vi "充电数据解析(81).vi"(1 "充电数据解析(81)":dbl[](array[numeric])) -> (0 "充电状态":string[](array[string]))   [LabVIEW 2013]
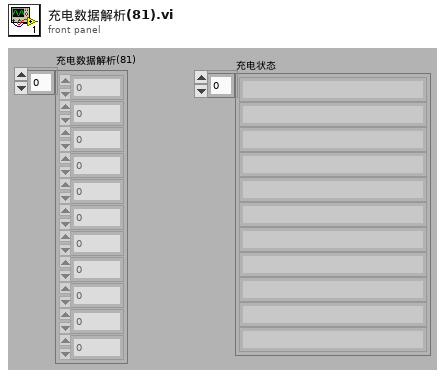
[diagram p1: front panel]
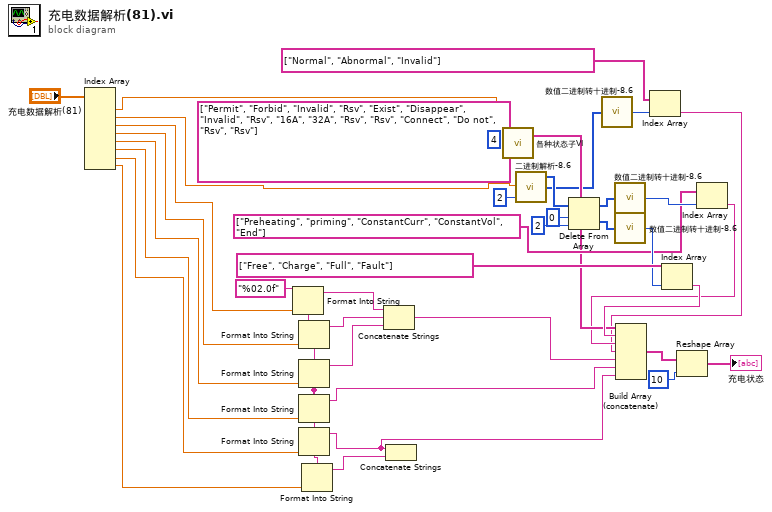
[diagram p0: block diagram]
diagram:
  w32 = "%02.0f" ("格式字符串")
  n1 = Index Array(array="充电数据解析(81)") -> (element #1=w12:dbl, element #2=w11:dbl, element #3=w10:dbl, element #4=w9:dbl, element #5=w8:dbl, element #6=w7:dbl, element #7=w6:dbl, element #8=w5:dbl)  [unwired: 8 in]
  n2 = Format Into String(format string=w32, w10) -> (resulting string=w33:string)  [unwired: 2 in, 1 out]
  n3 = Format Into String(format string=w32, w9) -> (resulting string=w34:string)  [unwired: 2 in, 1 out]
  n4 = Format Into String(format string=w32, w8) -> (resulting string=w35:string)  [unwired: 2 in, 1 out]
  n5 = Format Into String(format string=w32, w7) -> (resulting string=w38:string)  [unwired: 2 in, 1 out]
  n6 = Format Into String(format string=w32, w6) -> (resulting string=w39:string)  [unwired: 2 in, 1 out]
  n7 = Format Into String(format string=w32, w5) -> (resulting string=w36:string)  [unwired: 2 in, 1 out]
  n8 = Concatenate Strings(w33, w34, w35) -> (w37:string)
  n9 = Concatenate Strings(w39, w36) -> ()  [unwired: 1 out]
  n10 = call "各种状态子VI.vi"("状态输入"=string[][] [["Permit", "Forbid", "Invalid", "Rsv"], ["Exist", "Disappear", "Invalid", "Rsv"], ["16A", "32A", "Rsv", "Rsv"], ["Connect", "Do not", "Rsv", "Rsv"]], "几种类型"=4, "数值"=w12) -> ("状态"=w18:string[])  [unwired: 1 in, 1 out]
  n11 = call "二进制解析-8.6.vi"("索引"=2, "数值"=w11) -> ("低位子数组"=w4:i32[], "高位子数组"=w22:i32[])  [unwired: 2 out]
  n12 = Delete From Array(array=w22, length=0 ("长度"), index=2 ("索引")) -> (deleted portion=w25:i32[], array with subset deleted=w26:i32[])
  n13 = call "数值二进制转十进制-8.6.vi"("子数组"=w4) -> ("十进制数值"=w2:i32)  [unwired: 4 out]
  n14 = call "数值二进制转十进制-8.6.vi"("子数组"=w26) -> ("十进制数值"=w28:i32)  [unwired: 4 out]
  n15 = call "数值二进制转十进制-8.6.vi"("子数组"=w25) -> ("十进制数值"=w29:i32)  [unwired: 4 out]
  n16 = Index Array(array=string[] ["Normal", "Abnormal", "Invalid"] ("状态输入"), index=w2) -> (element=w1:string)
  n17 = Index Array(array=string[] ["Free", "Charge", "Full", "Fault"] ("状态输入"), index=w29) -> (element=w31:string)
  n18 = Index Array(array=string[] ["Preheating", "priming", "ConstantCurr", "ConstantVol", "End"] ("状态输入"), index=w28) -> (element=w15:string)
  n19 = Build Array (concatenate)(w18, w31, w15, w1, w37, w38, w39) -> (w19:string[])
  n20 = Reshape Array(w19, 10 ("维数大小")) -> (→"充电状态":string[])
